vi "Main.vi"(10 "JQMHStartup":refnum<class "RQMHStartup.lvclass">, 11 "NewTemplate in":refnum<class "ErrorHandler.lvclass">) -> ()   [LabVIEW 2024, in "ErrorHandler.lvclass"]
uses:
  ErrorHandler.lvclass
  C:/DevOps/CORTEX/JQMH/JQMHCore/Module/RQMHModule.lvclass
  JQMHCore/JQMHStartup/RQMHStartup.lvclass
  Message Queue_class/RQMHMessageQueue.lvclass/RQMHMessageQueue.ctl
  JQMHCore/Module/InitialiseReplyArgs.ctl
  <vilib>/Utility/miscctls.llb/LVPointTypeDef.ctl
  JQMHCore/Module/RQMHModule.lvclass/RQMHModule.ctl
  Do Something ReplyArgs.ctl
  Do Something Args.ctl
  JQMHCore/Module/Read ModuleName.vi
  JQMHCore/Module/Read External Start.vi
  Message Queue_class/Delacor_lib_QMH_Enqueue Message (Single).vi
  Message Queue_class/RQMHMessageQueue.lvclass
  ErrorHandler.lvclass/ErrorHandler.ctl
  JQMHCore/Module/RQMHModule.lvclass
  JQMHCore/Shared/JQMHShared.lvlib
panel:
  out "error out":errorcluster
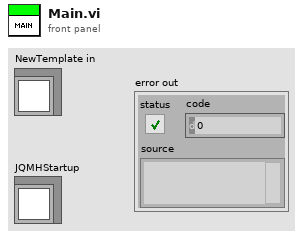
[diagram p1: front panel]
types:
  T1 = typedef "ErrorHandler.lvclass/Request Events--cluster.ctl" = cluster{"Do Something":refnum<user-event>}
  T2 = cluster{"Stop Module":refnum<user-event>, "Requests":T1}
  T3 = typedef "LVPointTypeDef.ctl" = cluster{"Horizontal":i16, "Vertical":i16}
  T4 = enum32{"Invalid", "Standard", "Closed", "Hidden", "Minimized", "Maximized"}
  T5 = typedef "RQMHModule.lvclass/InitialiseReplyArgs.ctl" = cluster{"Did Init?":bool}
  T6 = typedef "ErrorHandler.lvclass/Do Something Args.ctl" = cluster{"Msg":string}
  T7 = typedef "ErrorHandler.lvclass/Do Something ReplyArgs.ctl" = cluster{"Value":dbl, "Boolean":bool}
  T8 = typedef "RQMHModule.lvclass/Reply.ctl" = cluster{"Expects Reply":bool, "Reply":refnum<notifier>}
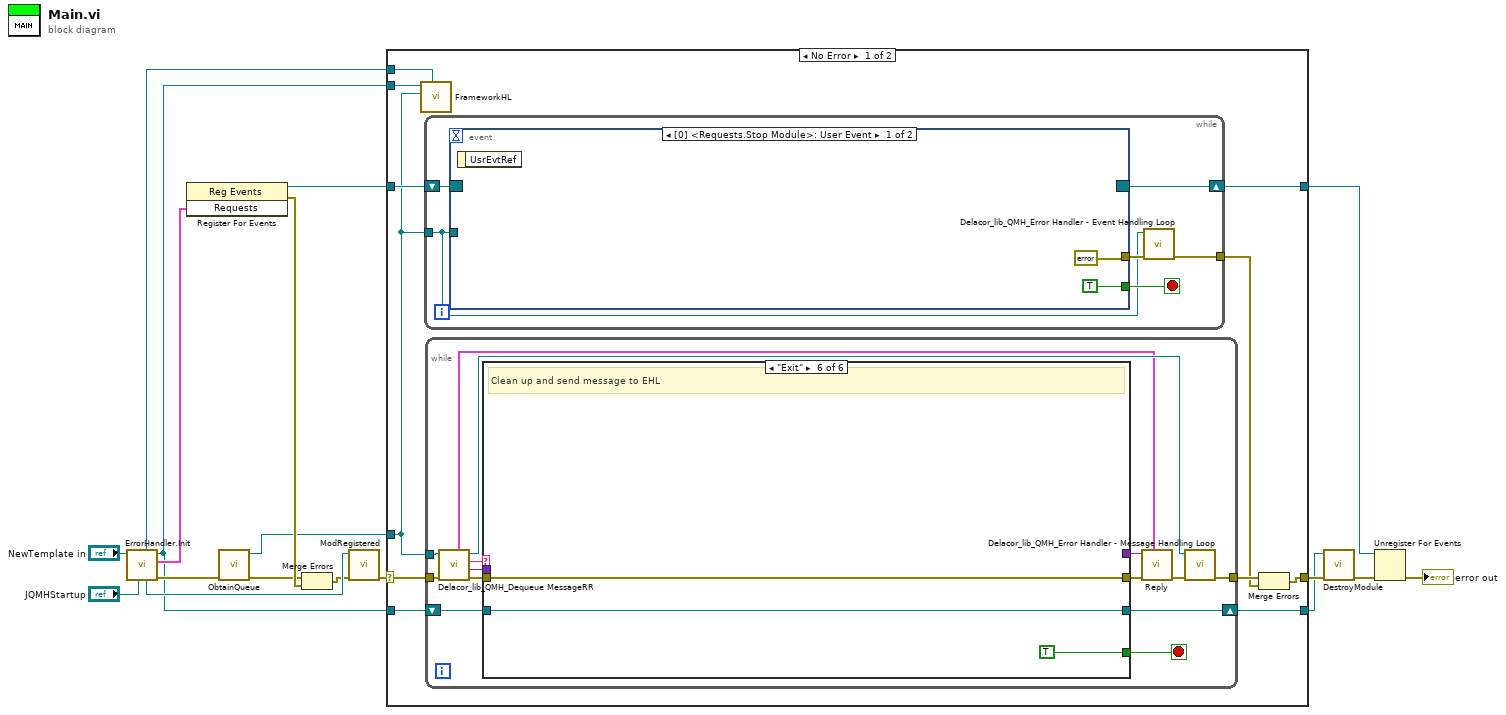
[diagram p0: block diagram]
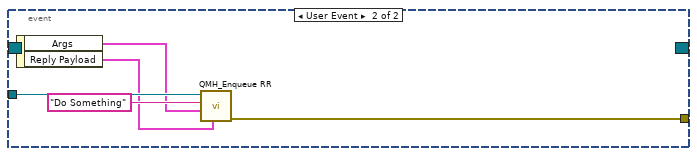
[diagram p2: hidden frame]
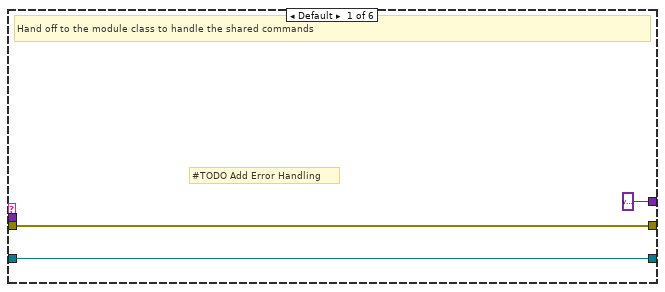
[diagram p3: hidden frame]
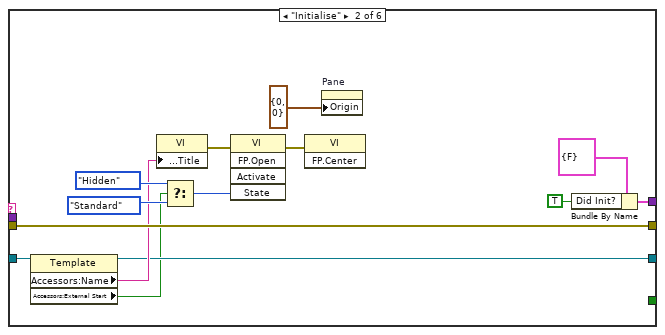
[diagram p4: hidden frame]
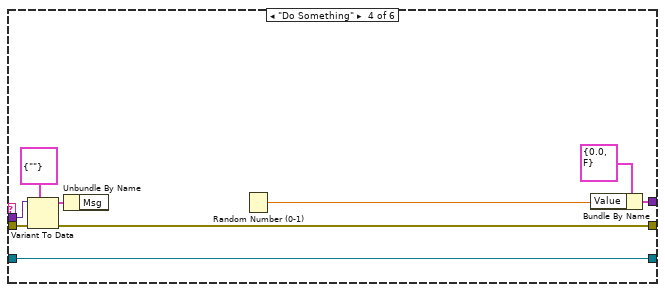
[diagram p6: hidden frame]
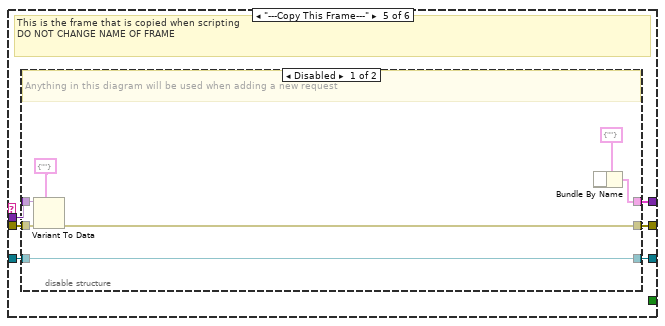
[diagram p7: hidden frame]
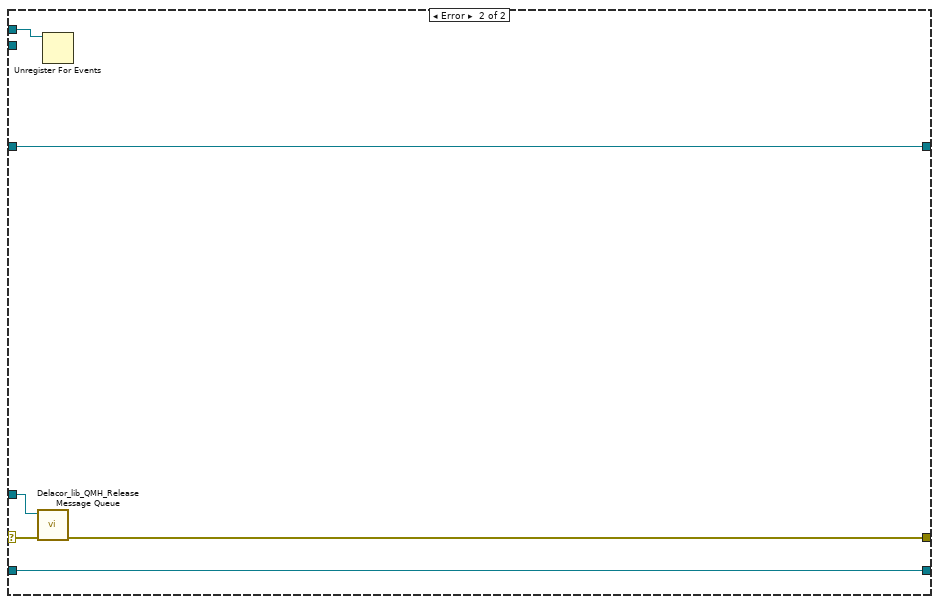
[diagram p9: hidden frame]
diagram:
  n1 = call "ErrorHandler.Init.vi"("JQMHStartup in"="JQMHStartup", "NewTemplate in"="NewTemplate in") -> ("error out"=w11:errorcluster, "Requests"=w2:T2, "NewTemplate out"=w1:refnum<class "ErrorHandler.lvclass">, "JQMHStartup out"=w9:refnum<class "RQMHStartup.lvclass">, "StandardRequests"=w5:refnum<event-registration>)  [unwired: 4 in, 1 out]
  n2 = register-events(w2) -> (reference out=w4:refnum<event-registration>, error out=w18:errorcluster)  [unwired: 2 in]
  n3 = call "ObtainQueue.vi"("error in"=w11) -> ("error out"=w10:errorcluster, "Message Queue"=w6:refnum<class "RQMHMessageQueue.lvclass">)  [unwired: 9 in]
  n4 = Merge Errors(w10, w18) -> (w7:errorcluster)
  n5 = call "ModRegistered.vi"("error in (no error)"=w7, "JQMHStartup in"=w9) -> ("error out"=w8:errorcluster)  [unwired: 9 in]
  n6 = case "RQMH_MAIN" shown="No Error" w8 {
    selector: w8 -> [w26 w106]
    tunnel: w1 -> [w29 w105]
    tunnel: [w28 w108] -> w17
    tunnel: w4 -> [w27 w108]
    tunnel: w6 -> [w20 w107]
    tunnel: [w25 w105] -> w3
    tunnel: [w22 w104] -> w14
    tunnel: w1 -> [w21 _]
    tunnel: w5 -> [w19 w103]
    frame No Error {
      n7 = call-dynamic "FrameworkHL.vi"("StandardRequests"=w19, "Message Queue"=w20, "JQMHModule in"=w21) -> ()  [unwired: 9 in]
      n8 = while {
        shift-right: [w35] -> w28
        shift-left: w27 -> [w30]
        tunnel: w20 -> [w31]
        tunnel: [w32] -> w23
        stop <- w34 stop-if-true
        n9 = event "RQMH_EVENT_MAIN" shown="[0] <Requests.Stop Module>: User Event" {
          selector: w30 -> [_ _]
          dyn-events: [_ _] -> w35
          timeout: _ -> [_ _]
          tunnel: [TRUE _] -> w34
          tunnel: w31 -> [_ w42]
          tunnel: [errorcluster {"status"=FALSE, "code"=0, "source"=""} ("error out") w39] -> w33
          event User Event {
            n10 = event-data() -> ()  [unwired: 1 in, 1 out]
          }
          event User Event {
            n11 = event-data() -> ("Args"=w40:T6, "Reply Payload"=w38:T8)  [unwired: 1 in]
            n12 = call "QMH_Enqueue RR.vi"("Reply"=w38, "Message Data"=w40, "Message"="Do Something", "Message Queue in"=w42) -> ("error out"=w39:errorcluster)  [unwired: 6 in, 1 out]
          }
        }
        n13 = call-dynamic "Delacor_lib_QMH_Error Handler - Event Handling Loop.vi"("error in"=w33, "Message Queue in"=w31) -> ("dup error in"=w32:errorcluster)  [unwired: 8 in, 1 out]
      }
      n14 = while {
        tunnel: w20 -> [w51]
        tunnel: w26 -> [w50]
        shift-right: [w53] -> w25
        shift-left: w29 -> [w54]
        tunnel: [w52] -> w24
        stop <- w56 stop-if-true
        n15 = call-dynamic "Delacor_lib_QMH_Dequeue MessageRR.vi"("error in"=w50, "Message Queue in"=w51) -> ("error out"=w49:errorcluster, "Message Data"=w47:variant, "Message"=w48:string, "Message Queue out"=w55:refnum<class "RQMHMessageQueue.lvclass">, "Reply"=w43:T8)  [unwired: 5 in]
        n16 = case "RQMH_MESSAGE_CASES" shown="\"Exit\"" w48 {
          tunnel: [_ _ _ _ _ TRUE] -> w56
          tunnel: w54 -> [w58 w61 w74 w84 w88 w101]
          tunnel: w47 -> [_ _ _ w80 w86 _]
          tunnel: w49 -> [w59 w73 w75 w79 w90 w100]
          tunnel: [w59 w73 w75 w78 w89 w100] -> w46
          tunnel: [w58 w62 w74 w84 w87 w101] -> w53
          tunnel: [variant w72 _ w83 w85 _] -> w44
          frame Default {
            # "#TODO Add Error Handling"
            # "Hand off to the module class to handle the shared commands"
          }
          frame "Initialise" {
            n17 = property class="Template"(reference=w61) -> (reference out=w62:refnum<class "ErrorHandler.lvclass">, "Accessors:Name"=w63:string, "Accessors:External Start"=w60:bool)  [unwired: 1 in, 1 out]
            n18 = property on="Property Node" class="VI"("Front Panel.Title"=w63) -> (error out=w70:errorcluster)  [unwired: 2 in, 1 out]
            n19 = Select(t=T4."Hidden" ("State"), s=w60, f=T4."Standard" ("State")) -> (s? t:f=w66:T4)
            n20 = invoke on="Invoke Node" class="VI" method="FP.Open"(error in=w70, "State"=w66) -> (error out=w69:errorcluster)  [unwired: 3 in, 4 out]
            n21 = invoke on="Invoke Node" class="VI" method="FP.Center"(error in=w69) -> ()  [unwired: 2 in, 3 out]
            n22 = property on="Pane" class="Pane"("Origin"=T3 {"Horizontal"=0, "Vertical"=0}) -> ()  [unwired: 2 in, 2 out]
            n23 = Bundle By Name(cluster=T5 {"Did Init?"=FALSE} ("Args"), "Did Init?"=TRUE) -> (w72:T5)
          }
          frame "---Module Specific---" {
          }
          frame "Do Something" {
            n24 = Variant To Data(error in=w79, type=T6 {"Msg"=""} ("Do Something Args"), Variant=w80) -> (data=w76:T6, error out=w78:errorcluster)
            n25 = Unbundle By Name(w76) -> ()  [unwired: 1 out]
            n26 = Random Number (0-1)() -> (number: 0 to 1=w81:dbl)
            n27 = Bundle By Name(cluster=T7 {"Value"=0.0, "Boolean"=FALSE}, "Value"=w81) -> (w83:T7)
          }
          frame "---Copy This Frame---" {
            # "This is the frame that is copied when scripting\nDO NOT CHANGE NAME OF FRAME"
            n28 = disable-structure shown="Disabled" {
              disable-tunnel: w90 -> [w94 w99]
              disable-tunnel: [w95 w99] -> w89
              disable-tunnel: w88 -> [w97 w98]
              disable-tunnel: [w97 w98] -> w87
              disable-tunnel: w86 -> [w96 _]
              disable-tunnel: [w92 _] -> w85
              frame Disabled {
                # "Anything in this diagram will be used when adding a new request"
                n29 = Variant To Data(error in=w94, type=cluster{string} {""} ("RQMH_MHL_MSG_PL"), Variant=w96) -> (error out=w95:errorcluster)  [unwired: 1 out]
                n30 = Bundle By Name(cluster=cluster{string} {""} ("RQMH_MHL_REPLY_PL")) -> (w92:cluster{string})  [unwired: 1 in]
              }
              frame Enabled {
              }
            }
          }
          frame "Exit" {
            # "Clean up and send message to EHL"
          }
        }
        n31 = call "Reply.vi"("Reply"=w43, "error in (no error)"=w46, "ReplyPayload"=w44) -> ("error out"=w45:errorcluster)  [unwired: 8 in]
        n32 = call-dynamic "Delacor_lib_QMH_Error Handler - Message Handling Loop.vi"("error in"=w45, "Message Queue in"=w55) -> ("dup error in"=w52:errorcluster)  [unwired: 8 in, 1 out]
      }
      n33 = Merge Errors(w24, w23) -> (w22:errorcluster)
    }
    frame Error {
      n34 = call-dynamic "Delacor_lib_QMH_Release Message Queue.vi"("error in"=w106, "Message Queue"=w107) -> ("error out"=w104:errorcluster)  [unwired: 9 in]
      n35 = Unregister For Events(event registration refnum=w103) -> ()  [unwired: 1 in, 1 out]
    }
  }
  n36 = call "DestroyModule.vi"("error in (no error)"=w14, "JQMHModule in"=w3) -> ("error out"=w16:errorcluster)  [unwired: 9 in]
  n37 = Unregister For Events(event registration refnum=w17, error in=w16) -> (error out=→"error out":errorcluster)
